vi "Get Vehicle Pose.vi"(8 "error in (no error)":errorcluster, 11 "Simulator in":refnum<class "Simulator.lvclass">) -> (0 "error out":errorcluster, 1 "Vehicle Bearing (rads)":dbl, 2 "Vehicle Location":cluster{"x":dbl, "y":dbl}, 3 "Simulator out":refnum<class "Simulator.lvclass">)   [LabVIEW 2011, in "Simulator.lvclass"]
uses:
  Simulator.lvclass
  Simulator.lvclass/Simulator.ctl
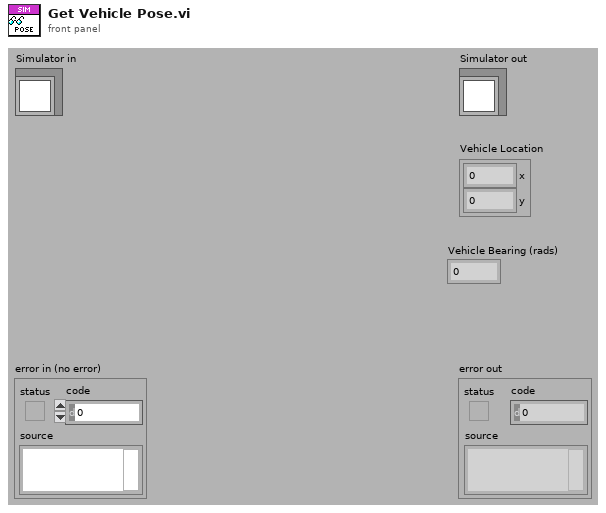
[diagram p1: front panel]
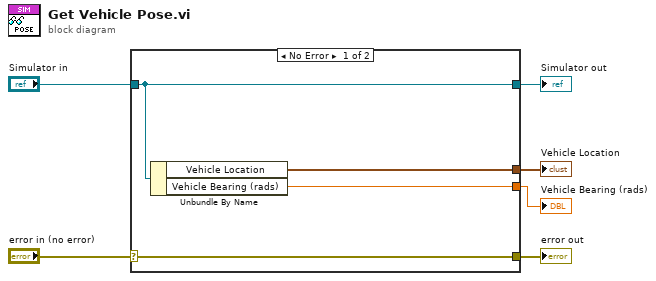
[diagram p0: block diagram]
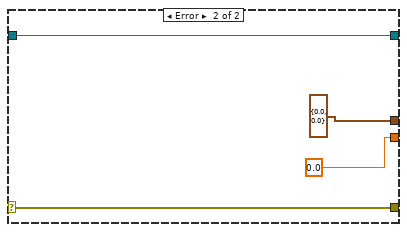
[diagram p2: hidden frame]
diagram:
  n1 = case shown="No Error" "error in (no error)" {
    selector: "error in (no error)" -> [w10 w13]
    tunnel: [w10 w13] -> w5
    tunnel: [w9 w14] -> w3
    tunnel: "Simulator in" -> [w9 w14]
    tunnel: [w8 cluster{"x":dbl, "y":dbl} {"x"=0.0, "y"=0.0} ("Vehicle Location")] -> w2
    tunnel: [w7 0.0 ("Vehicle Bearing (rads)")] -> w1
    frame No Error {
      n2 = Unbundle By Name(w9) -> ("Vehicle Location"=w8:cluster{"x":dbl, "y":dbl}, "Vehicle Bearing (rads)"=w7:dbl)
    }
    frame Error {
    }
  }
  "error out" <- w5
  "Simulator out" <- w3
  "Vehicle Location" <- w2
  "Vehicle Bearing (rads)" <- w1
